vi "C8855-01_Close.vi"(8 "MainD":T1 {"G_DIM" format="%.5f"}, 11 "Continue":bool) -> ()   [LabVIEW 2017]
uses:
  C8855_MainD.ctl
  C8855-01api.dll
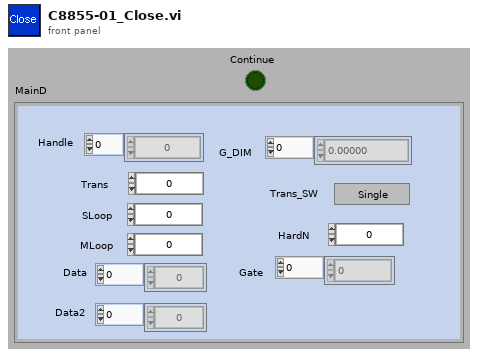
[diagram p1: front panel]
types:
  T1 = typedef "C8855_MainD.ctl" = cluster{"Handle":i64[], "G_DIM":dbl[], "Trans":u16, "Trans_SW":bool, "HardN":i32, "Gate":u8[], "Data":u32[], "Data2":u32[], "SLoop":i32, "MLoop":i32}
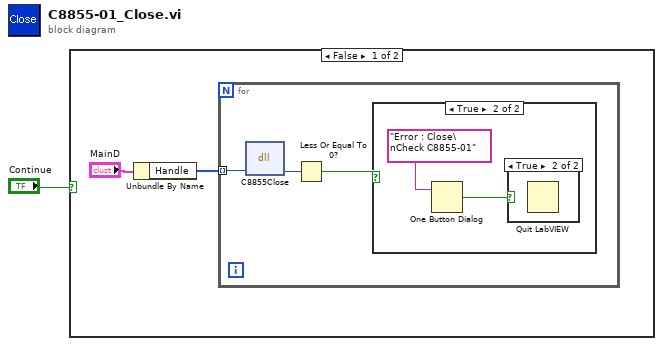
[diagram p0: block diagram]
diagram:
  n1 = case shown="False" "Continue" {
    frame False {
      n2 = Unbundle By Name("MainD") -> ("Handle"=w2:i64[])
      n3 = for {
        tunnel: w2 -> [w6] mode=indexing
        n4 = dll-call lib="C:/Users/PC33412/Desktop/CD_Ver3.3.0/Sample/Source/x64/C8855-01api.dll" fn="C8855Close"("Handle"=w6) -> ("Handle"=w5:i64)  [unwired: 3 in, 3 out]
        n5 = Less Or Equal To 0?(x=w5) -> (x <= 0?=w4:bool)
        n6 = case shown="True" w4 {
          frame False {
          }
          frame True {
            n7 = One Button Dialog(message="Error : Close\nCheck C8855-01" ("爷景嫁")) -> (true=w7:bool)  [unwired: 1 out]
            n8 = case shown="True" w7 {
              frame False {
              }
              frame True {
                n9 = Quit LabVIEW() -> ()  [unwired: 1 out]
              }
            }
          }
        }
      }
    }
    frame True {
    }
  }
